vi "calcLoopTime.vi"(8 "error in (no error)":errorcluster, 11 "ComponentData in":refnum<class "ComponentData.lvclass">) -> (0 "error out":errorcluster, 3 "ComponentData out":refnum<class "ComponentData.lvclass">)   [LabVIEW 2013, in "ComponentData.lvlib" / "ComponentData.lvclass"]
uses:
  <userlib>/Common/Component/Application/RT/ComponentData/ComponentData/ComponentData.lvclass
  <userlib>/Common/Component/Application/RT/ComponentData/ComponentData/ComponentData.lvclass/ComponentData.ctl
  <userlib>/Common/Component/Application/RT/ComponentData/LoopTimer/LoopTimer.lvclass
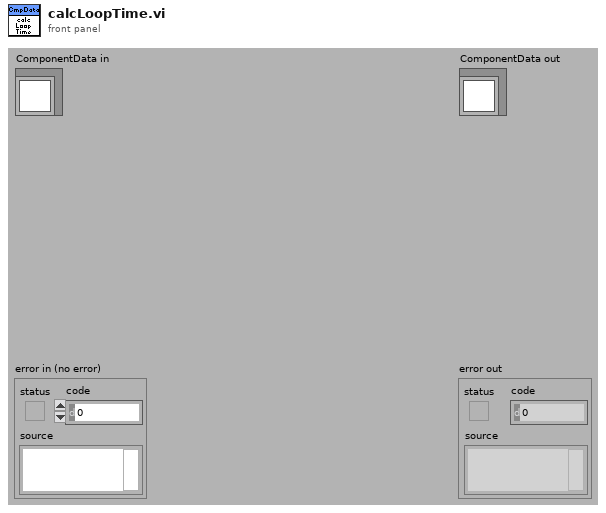
[diagram p1: front panel]
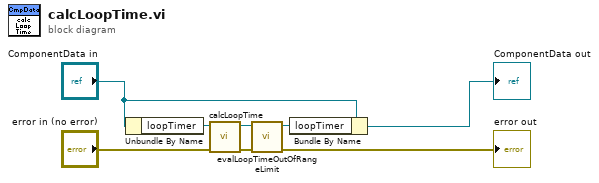
[diagram p0: block diagram]
diagram:
  n1 = Unbundle By Name("ComponentData in") -> ("loopTimer"=w4:refnum<class "LoopTimer.lvclass">)
  n2 = call <userlib>:"calcLoopTime.vi"("error in (no error)"="error in (no error)", "LoopTimer in"=w4) -> ("error out"=w1:errorcluster, "LoopTimer out"=w3:refnum<class "LoopTimer.lvclass">)  [unwired: 8 in]
  n3 = call <userlib>:"evalLoopTimeOutOfRangeLimit.vi"("error in (no error)"=w1, "LoopTimer in"=w3) -> ("error out"=→"error out":errorcluster, "LoopTimer out"=w2:refnum<class "LoopTimer.lvclass">)  [unwired: 8 in]
  n4 = Bundle By Name(cluster="ComponentData in", "loopTimer"=w2) -> (→"ComponentData out":refnum<class "ComponentData.lvclass">)
